vi "Update after ProtocollParameter Changes.vi"(0 "EPA Auswertung (Eingang)":refnum<vi>, 5 "Lin-Polynom":T1 {"zusätzliche Zeitdauer Erster Punkt" format="%#_5g"; "Lin Modus" items=["Cal Gas to PNS", "Cal Gas to Samplepoint", "Measure"]; "Gas Ablaufdatum" format="%<%d.%m.%Y>T"; "HovaCAL Flow AutoLin"."HovaCAL Flow Input Cluster" format="%.2f"; "Gasflasche" items=["----"=10000, "IAG MG"=0, "IAG NH3 3000"=1, "IAG NH3 2000"=2, "IAG NH3 200"=3]; "Conditions:" items=["field", "laboratory"]; "Kalibrierauswahl" items=["Inaktiv", "Aktiv"]; "Anzahl Stufen" format="%#_5g"; "Zeitdauer Stufe" format="%#_5g"; "Verdünnungsgas" items=["N2", "O2"]; "Komponentenauswahl"."Konzentration" format="%#.6f"; "Gasnummer:" min=1 max=5; "Prüfgas Konzentration" format="%#.6f"; "Polynomkoeff." format="%#_18f"}, 7 "Polynom-Ordnung (Eingang)":refnum<vi>, 11 "Fehler (Eingang)":errorcluster caption="Fehler (Eingang, kein Fehler)") -> (2 "Aktiv EPA":T15, 3 "Stufen Tabelle":T18, 4 "Polynomkoeff.":T17, 6 "EPA Ausgabetabelle":string[][](array[string]), 8 "LIN Ausgabetabelle":string[][](array[string]), 10 "XY-Graph":cluster{dbl[], dbl[]}[](array[cluster]), 13 "Formel":string, 14 "LINVer Auswertung":string[][](array[string]), 15 "Fehler (Ausgang)":errorcluster)   [LabVIEW 2020, in "Linearisierung v2.lvlib" / "SpanEinstellungen.lvlib"]
uses:
  SpanEinstellungen/SpanEinstellungen.lvlib
  Gasteiler/Stufen Tabelle.ctl
  AktivArray.ctl
  AktivButton.ctl
  Lin-Polynom Daten.ctl
  KomponentenArray.ctl
  Visualisierungs Elemente/Auswahlfeld.ctl
  Visualisierungs Elemente/Zahlen-Eingabefeld.ctl
  EPA Optionsfeld.ctl
  Gasteiler/HovaCal/AutoLin Hovacal.ctl
  Kalibrieroption.ctl
  EPA1065-307/Condition.ctl
  Seiten/System Einstellungen V2/Konfig Gasflasche.ctl
  Seiten/System Einstellungen V2/Gasflasche Auswahl.ctl
  Gasteiler/HovaCAL_Interface/Controls/Flow Einstellung.ctl
  Gasteiler/HovaCAL_Interface/Controls/Pump state.ctl
  Seiten/CalGas Aufschaltung/Lin Modus.ctl
  Aktion Lin Daten aufarbeiten.ctl
  Gasteiler/Aktion FGV Gasteilerliste laden.ctl
  EPA1065-307/Aktion FGV Auswertung sammeln.ctl
  Linearisierung v2.lvlib
  Gasteiler/Gasteiler.lvlib
  EPA1065-307/Linearity verification 1065-307.lvlib
  Gasteiler/HovaCal/HovaCal.lvlib
  Seiten/System Einstellungen V2/System Einstellungen V2.lvlib
  Gasteiler/HovaCAL_Interface/Controls/Controls.lvlib
  Seiten/CalGas Aufschaltung/CalGas Aufschaltung.lvlib
panel:
  # "%"
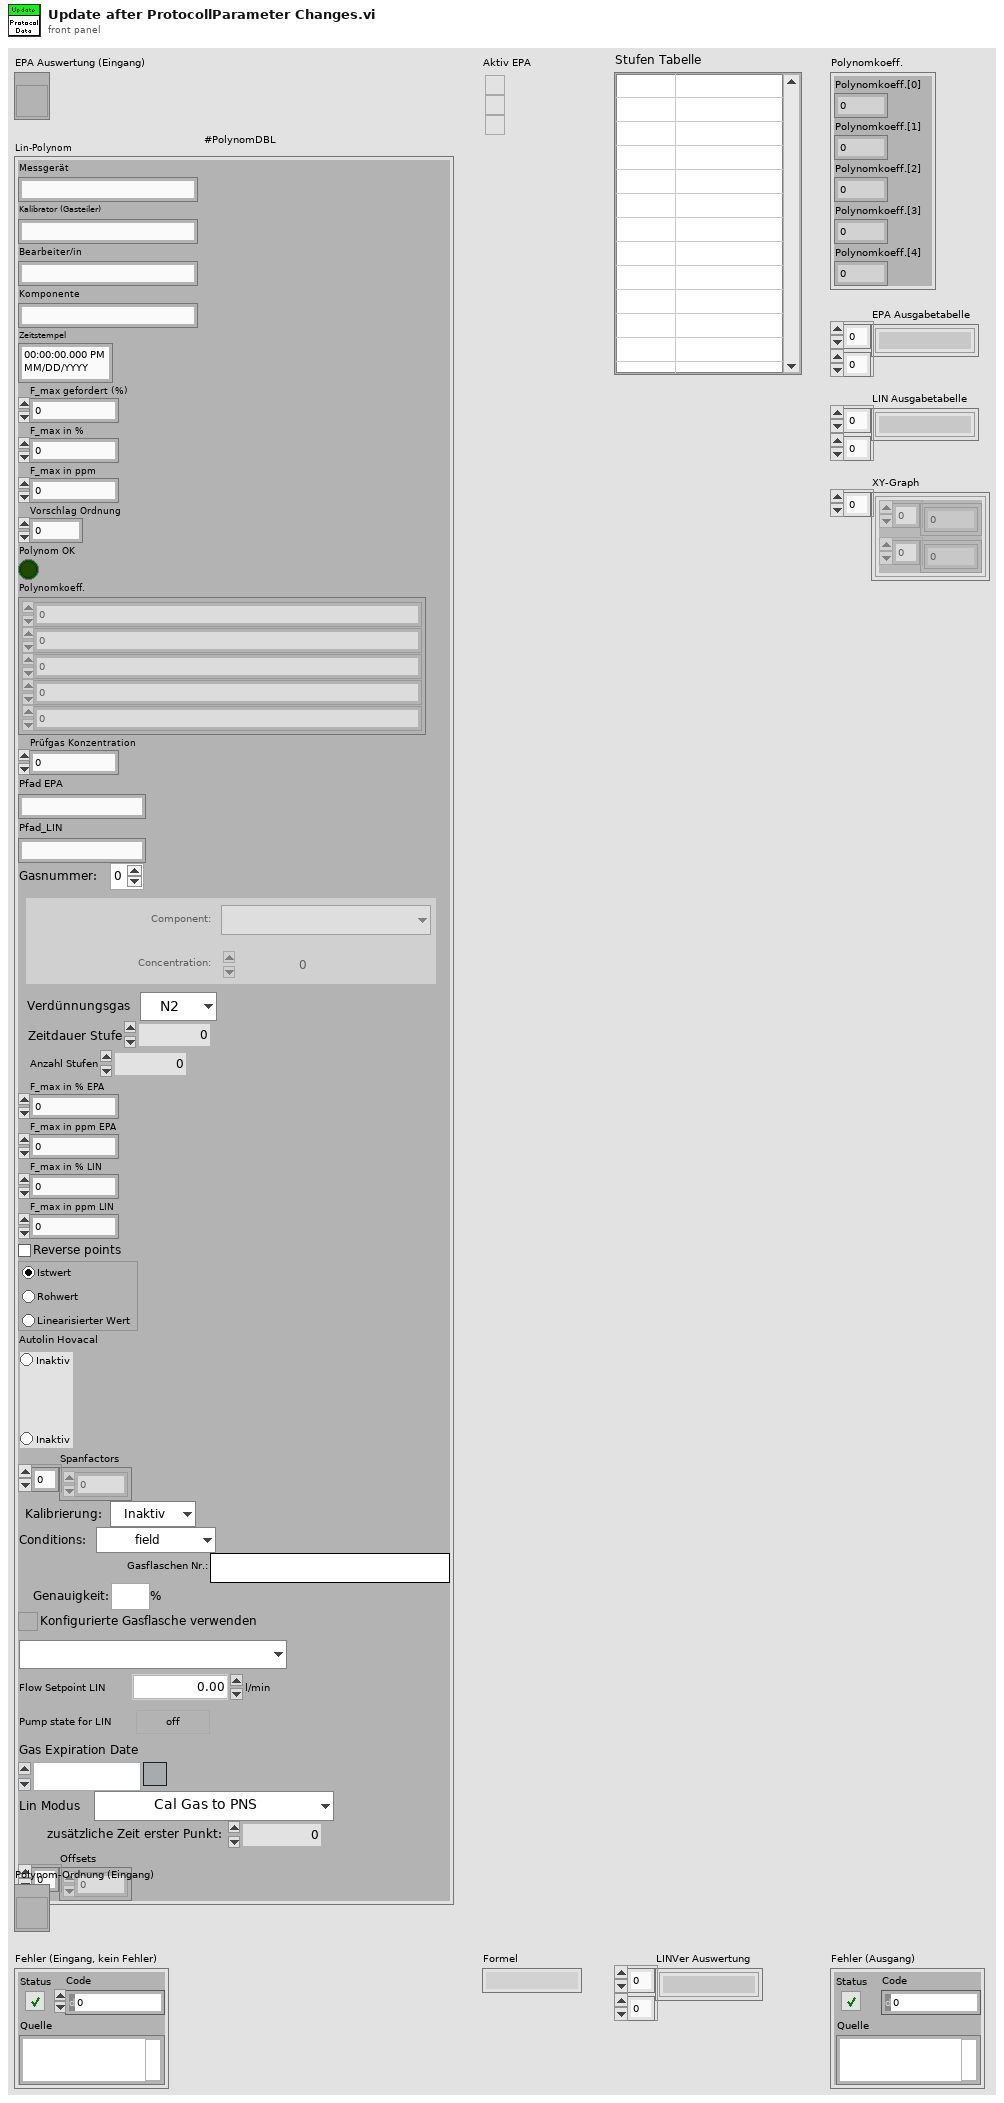
[diagram p1: front panel]
types:
  T1 = typedef "Linearisierung v2.lvlib/Lin-Polynom Daten.ctl" = cluster{"Messgerät":string, "Kalibrator (Gasteiler)":string, "Bearbeiter/in":string, "Komponente":string, "Zeitstempel":timestamp, "F_max gefordert (%)":sgl, "F_max in %":sgl, "F_max in ppm":sgl, "Vorschlag Ordnung":i32, "Polynom OK":bool, "Polynomkoeff.":dbl[], "Prüfgas Konzentration":dbl, "Pfad EPA":string, "Pfad_LIN":string, "Gasnummer:":u8, "Komponentenauswahl":T2, "Verdünnungsgas":T4, "Zeitdauer Stufe":T5, "Anzahl Stufen":T5, "F_max in % EPA":sgl, "F_max in ppm EPA":sgl, "F_max in % LIN":sgl, "F_max in ppm LIN":sgl, "Punkte umkehren":bool, "EPA Optionsfeld":T6, "Autolin Hovacal":T7, "Spanfactors":sgl[], "Kalibrierauswahl":T8, "Conditions:":T9, "Gasflaschen Nr.:":string, "Bottle Accuracy":dbl, "Konfig Gasflasche":T10, "Gasflasche":T11, "HovaCAL Flow AutoLin":T12, "MFC Output":T13, "Gas Ablaufdatum":timestamp, "Lin Modus":T14, "zusätzliche Zeitdauer Erster Punkt":sgl, "Offsets":sgl[]}
  T2 = typedef "Linearisierung v2.lvlib/KomponentenArray.ctl" = cluster{"Komponente:":T3, "Konzentration":dbl}[]
  T3 = typedef "Auswahlfeld.ctl" = u16
  T4 = typedef "Linearisierung v2.lvlib/Gasteiler.lvlib/Prüfgas in.ctl" = u16
  T5 = typedef "Zahlen-Eingabefeld.ctl" = sgl
  T6 = typedef "Linearisierung v2.lvlib/EPA Optionsfeld.ctl" = enum32{"Istwert", "Rohwert", "Linearisierter Wert"}
  T7 = typedef "Linearisierung v2.lvlib/Gasteiler.lvlib/HovaCal.lvlib/AutoLin Hovacal.ctl" = enum32{"Keine Auswahl", "Optionsauswahl 1", "Optionsauswahl 2"}
  T8 = typedef "Linearisierung v2.lvlib/Kalibrieroption.ctl" = u16
  T9 = typedef "Linearisierung v2.lvlib/Linearity verification 1065-307.lvlib/Condition.ctl" = u16
  T10 = typedef "System Einstellungen V2.lvlib/Konfig Gasflasche.ctl" = bool
  T11 = typedef "System Einstellungen V2.lvlib/Gasflasche Auswahl.ctl" = u16
  T12 = typedef "Linearisierung v2.lvlib/Gasteiler.lvlib/HovaCAL_Interface.lvlib/Controls.lvlib/Flow Einstellung.ctl" = cluster{"HovaCAL Flow Input Cluster":dbl}
  T13 = typedef "Linearisierung v2.lvlib/Gasteiler.lvlib/HovaCAL_Interface.lvlib/Controls.lvlib/Pump state.ctl" = cluster{"Run":bool}
  T14 = typedef "CalGas Aufschaltung.lvlib/Lin Modus.ctl" = u16
  T15 = typedef "Linearisierung v2.lvlib/AktivArray.ctl" = T16[]
  T16 = typedef "Linearisierung v2.lvlib/AktivButton.ctl" = bool
  T17 = cluster{"Polynomkoeff.[0]":sgl, "Polynomkoeff.[1]":sgl, "Polynomkoeff.[2]":sgl, "Polynomkoeff.[3]":sgl, "Polynomkoeff.[4]":sgl}
  T18 = typedef "Linearisierung v2.lvlib/Gasteiler.lvlib/Stufen Tabelle.ctl" = string[][]
  T19 = typedef "Linearisierung v2.lvlib/Aktion Lin Daten aufarbeiten.ctl" = enum16{"lesen", "Protkolldaten", "speichern", "laden", "EPA auswerten", "Tabelle schreiben", "Lin auswerten", "Tab init", "Stufentabelle", "EPA aktiviert", "Nachbehandlung laden", "Tabelle löschen", "Istwerte löschen", "Zeile löschen", "Zeile einfügen", "LIN aktiviert", "LIN/EPA aktiv laden", "EGAK Tab", "LIN übernehmen", "Tab init ohne Stufen"}
  T20 = typedef "Linearisierung v2.lvlib/Linearity verification 1065-307.lvlib/Aktion FGV Auswertung sammeln.ctl" = enum16{"lesen", "Auswertung", "löschen"}
  T21 = typedef "Linearisierung v2.lvlib/Gasteiler.lvlib/Aktion FGV Gasteilerliste laden.ctl" = enum16{"lesen", "laden", "speichern", "Liste erstellen", "Formel ändern", "Gas vereinzeln"}
  T22 = typedef "Linearisierung v2.lvlib/Auswahl Polynom Ordnung.ctl" = enum16{"autom.", "raw", "actual", "1", "2", "3", "4"}
  T23 = typedef "Linearisierung v2.lvlib/Eingabetabelle.ctl" = string[][]
  T24 = cluster{"Polynomkoeff.[0]":dbl, "Polynomkoeff.[1]":dbl, "Polynomkoeff.[2]":dbl, "Polynomkoeff.[3]":dbl, "Polynomkoeff.[4]":dbl}
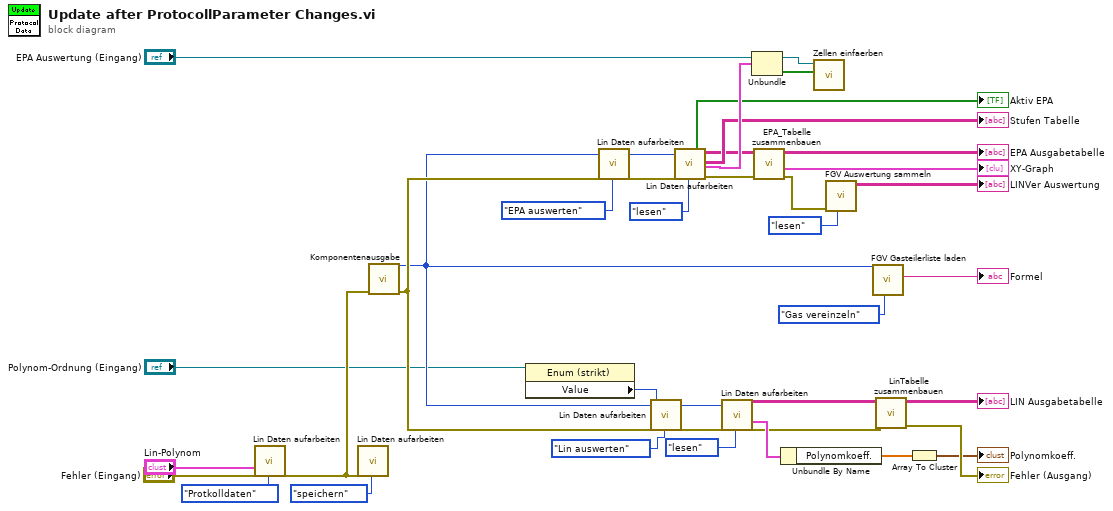
[diagram p0: block diagram]
diagram:
  n1 = call "Lin Daten aufarbeiten.vi"("Lin-Polynom"="Lin-Polynom", "error in (no error)"="Fehler (Eingang)", "Aktionen"=Aktion_Lin_Daten_aufarbeiten."Protkolldaten") -> ("error out"=w34:errorcluster)  [unwired: 14 in, 10 out]
  n2 = call "Lin Daten aufarbeiten.vi"("error in (no error)"=w34, "Aktionen"=Aktion_Lin_Daten_aufarbeiten."speichern") -> ()  [unwired: 15 in, 11 out]
  n3 = call "Komponentenausgabe.vi"("error in (no error)"=w34) -> ("error out"=w35:errorcluster, "Gaskomponente"=w26:T3)  [unwired: 7 in, 2 out]
  n4 = property class="Enum (strikt)"(reference="Polynom-Ordnung (Eingang)") -> ("Value"=w23:T22)  [unwired: 1 in, 2 out]
  n5 = call "Lin Daten aufarbeiten.vi"("Index (Seite)"=w26, "error in (no error)"=w35, "Aktionen"=Aktion_Lin_Daten_aufarbeiten."EPA auswerten") -> ("Index (Seite) out"=w36:i32, "error out"=w10:errorcluster)  [unwired: 14 in, 9 out]
  n6 = call "Lin Daten aufarbeiten.vi"("Index (Seite)"=w26, "error in (no error)"=w35, "Polynom-Ordnung"=w23, "Aktionen"=Aktion_Lin_Daten_aufarbeiten."Lin auswerten") -> ("Index (Seite) out"=w37:i32, "error out"=w25:errorcluster)  [unwired: 13 in, 9 out]
  n7 = call "Lin Daten aufarbeiten.vi"("Index (Seite)"=w36, "error in (no error)"=w10, "Aktionen"=Aktion_Lin_Daten_aufarbeiten."lesen") -> ("Aktiv EPA"=→"Aktiv EPA":T15, "Eingabetabelle"=w8:T23, "Stufen Tabelle"=→"Stufen Tabelle":T18, "EPA Auswertung"=w33:cluster{sgl[], sgl[], bool[]}, "error out"=w9:errorcluster)  [unwired: 14 in, 6 out]
  n8 = call "Lin Daten aufarbeiten.vi"("Index (Seite)"=w37, "error in (no error)"=w25, "Aktionen"=Aktion_Lin_Daten_aufarbeiten."lesen") -> ("Eingabetabelle"=w19:T23, "Lin-Polynom"=w29:T1, "error out"=w21:errorcluster)  [unwired: 14 in, 8 out]
  n9 = Unbundle(w33) -> (w31:bool[])  [unwired: 2 out]
  n10 = call "EPA_Tabelle zusammenbauen.vi"("error in (no error)"=w9, "Eingabetabelle"=w8) -> ("error out"=w14:errorcluster, "XY-Graph"=→"XY-Graph":cluster{dbl[], dbl[]}[], "EPA Ausgabetabelle"=→"EPA Ausgabetabelle":string[][])  [unwired: 7 in]
  n11 = Unbundle By Name(w29) -> ("Polynomkoeff."=w28:dbl[])
  n12 = call "Zellen einfaerben.vi"("Färben"=w31, "Tabellenref."="EPA Auswertung (Eingang)") -> ()  [unwired: 10 in]
  n13 = call "FGV Auswertung sammeln.vi"("Aktion"=Aktion_FGV_Auswertung_sammeln."lesen", "error in (no error)"=w14) -> ("LINVer Auswertung"=→"LINVer Auswertung":string[][])  [unwired: 7 in, 2 out]
  n14 = call "FGV Gasteilerliste laden.vi"("Aktion"=Aktion_FGV_Gasteilerliste_laden."Gas vereinzeln", "Gasindex"=w26) -> ("Formel"=→"Formel":string)  [unwired: 7 in, 2 out]
  n15 = call "LinTabelle zusammenbauen.vi"("error in (no error)"=w21, "Eingabetabelle"=w19) -> ("error out"=→"Fehler (Ausgang)":errorcluster, "LIN Ausgabetabelle"=→"LIN Ausgabetabelle":string[][])  [unwired: 6 in, 2 out]
  n16 = Array To Cluster(array=w28) -> (cluster=→"Polynomkoeff.":T24)
